vi "Module Type.vi"(11 "Data Logger Module in":refnum<class "Data Logger DBL Module.lvclass">) -> (2 "Module Type":string)   [LabVIEW 2020, in "VolatusData.lvlib" / "Data Logger DBL Module.lvclass"]
uses:
  Data Logger DBL Module.lvclass
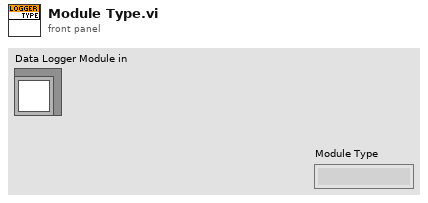
[diagram p1: front panel]
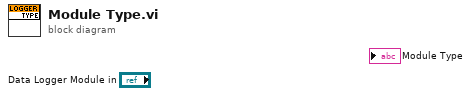
[diagram p0: block diagram]
diagram:
